vi "Control Dead zone.vi"(10 "dead zone":dbl, 11 "control Value":dbl) -> (2 "Active":bool, 3 "output Value":dbl)   [LabVIEW 2020]
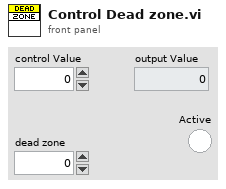
[diagram p1: front panel]
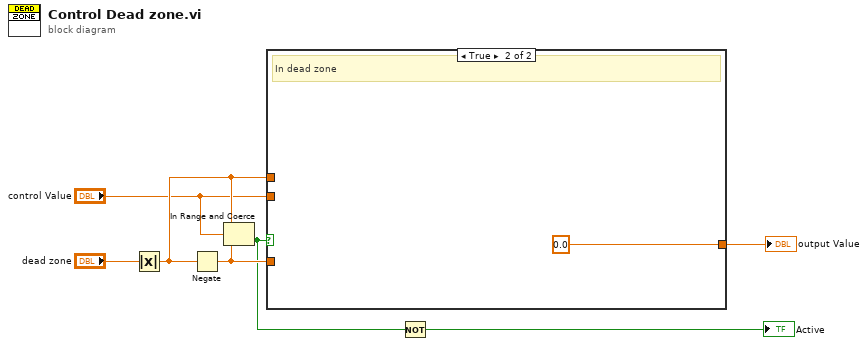
[diagram p0: block diagram]
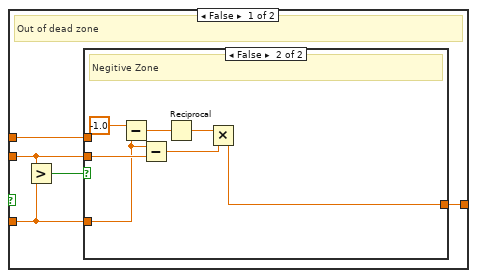
[diagram p2: hidden frame]
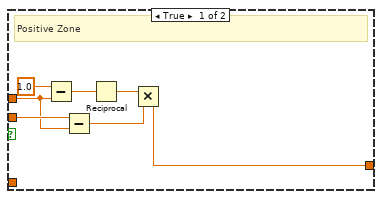
[diagram p3: hidden frame]
diagram:
  n1 = Absolute Value(x="dead zone") -> (abs(x)=w5:dbl)
  n2 = Negate(x=w5) -> (-x=w4:dbl)
  n3 = In Range and Coerce(upper limit=w5, x="control Value", lower limit=w4) -> (In Range?=w2:bool)  [unwired: 1 out]
  n4 = case shown="True" w2 {
    tunnel: "control Value" -> [w11 _]
    tunnel: [w8 0.0] -> w6
    tunnel: w5 -> [w10 _]
    tunnel: w4 -> [w9 _]
    frame False {
      # "Out of dead zone"
      n5 = Greater?(x=w11, y=w9) -> (0:w12:bool)
      n6 = case shown="False" w12 {
        tunnel: w11 -> [w17 w21]
        tunnel: w10 -> [w16 _]
        tunnel: w9 -> [_ w20]
        tunnel: [w13 w22] -> w8
        frame True {
          # "Positive Zone"
          n7 = Subtract(x=1.0, y=w16) -> (x-y=w18:dbl)
          n8 = Subtract(x=w17, y=w16) -> (x-y=w14:dbl)
          n9 = Reciprocal(x=w18) -> (1/x=w15:dbl)
          n10 = Multiply(x=w15, y=w14) -> (x*y=w13:dbl)
        }
        frame False {
          # "Negitive Zone"
          n11 = Subtract(x=-1.0, y=w20) -> (x-y=w25:dbl)
          n12 = Subtract(x=w20, y=w21) -> (x-y=w23:dbl)
          n13 = Reciprocal(x=w25) -> (1/x=w24:dbl)
          n14 = Multiply(x=w24, y=w23) -> (x*y=w22:dbl)
        }
      }
    }
    frame True {
      # "In dead zone"
    }
  }
  "output Value" <- w6
  n15 = Not(x=w2) -> (.not. x?=→"Active":bool)
